vi "Recalculation_Monitor - 3 SC.vi"(0 "Alpha":dbl(slide)=0.17500000000000002 step=0.005 scale=0.0..1.0, 1 "Message 1":string="Lorem ipsum dolor sit amet, consetetur sadipscing elitr, sed diam nonumy eirmod tempor invidunt ut labore et dolore magna aliquyam erat, sed diam volu", 2 "Message 2":string="ptua. At vero eos et accusam et justo duo dolores et ea rebum. Stet clita kasd gubergren, no sea takimata sanctus est Lorem ipsum dolor sit amet. Lore", 3 "Alpha old":dbl(slide)=0.17500000000000002 step=0.005 scale=0.0..1.0, 4 "Message 1 old":string="Lorem ipsum dolor sit amet, consetetur sadipscing elitr, sed diam nonumy eirmod tempor invidunt ut labore et dolore magna aliquyam erat, sed diam volu", 5 "Message 2 old":string="ptua. At vero eos et accusam et justo duo dolores et ea rebum. Stet clita kasd gubergren, no sea takimata sanctus est Lorem ipsum dolor sit amet. Lore", 6 "Beta/Alpha":dbl(slide)=0.17500000000000002 step=0.005 scale=0.0..1.0, 8 "Beta/Alpha old":dbl(slide)=0.17500000000000002 step=0.005 scale=0.0..1.0) -> (14 "Recalculate?":bool, 15 "Recalculate SIG":bool, 16 "Recalculate OFDM":bool)   [LabVIEW 2022 SP3]
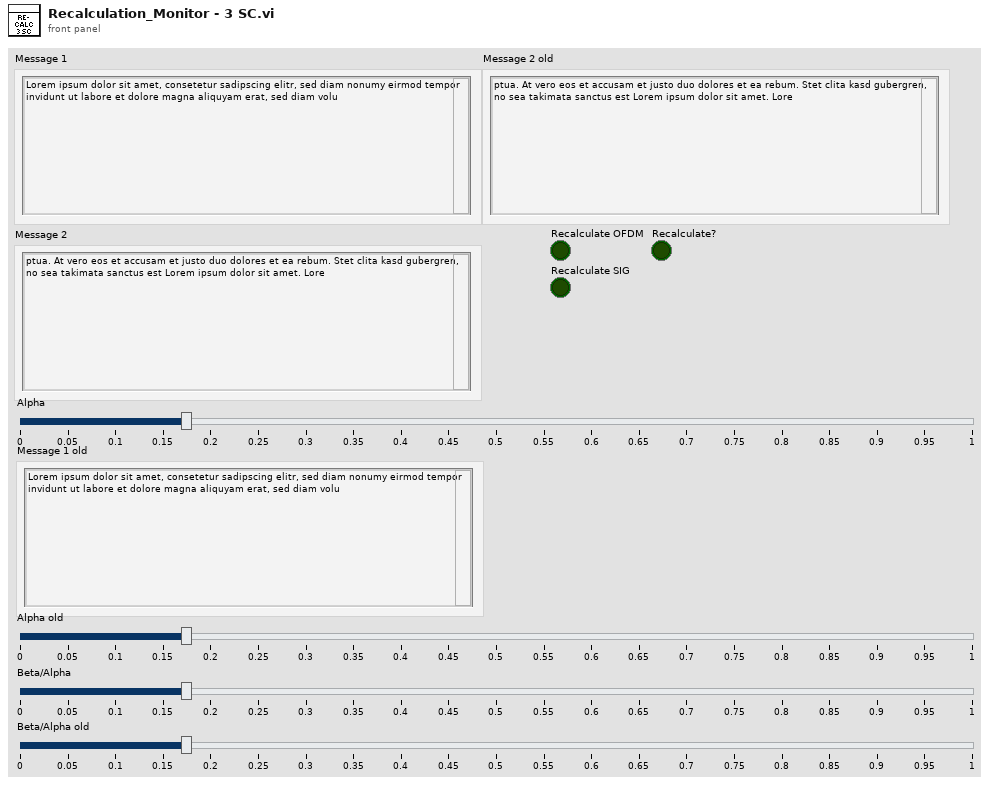
[diagram p1: front panel]
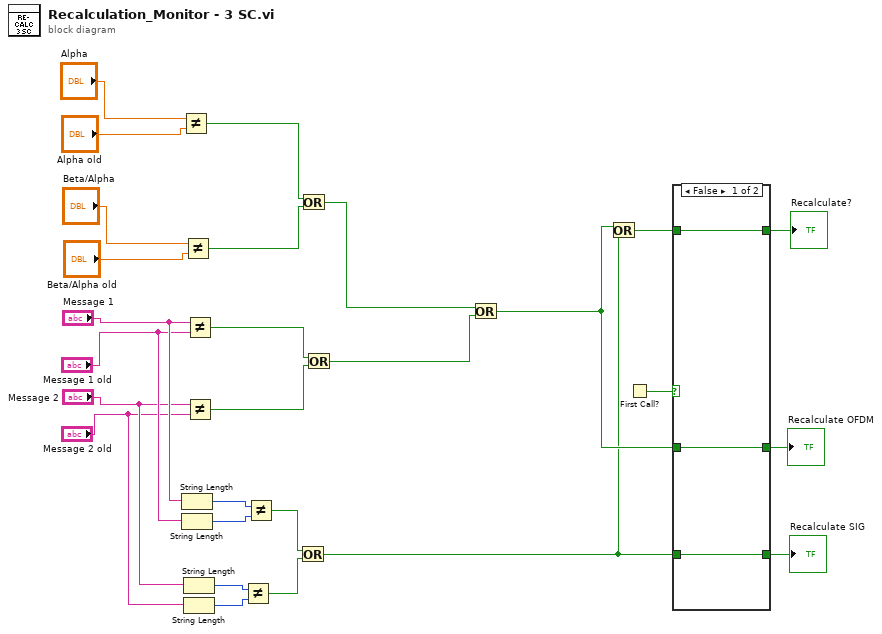
[diagram p0: block diagram]
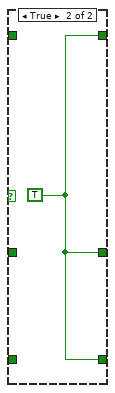
[diagram p2: hidden frame]
diagram:
  n1 = Not Equal?(x="Alpha", y="Alpha old") -> (x != y?=w3:bool)
  n2 = String Length(string="Message 1") -> (length=w19:i32)
  n3 = String Length(string="Message 1 old") -> (length=w18:i32)
  n4 = Not Equal?(x="Beta/Alpha", y="Beta/Alpha old") -> (x != y?=w2:bool)
  n5 = String Length(string="Message 2") -> (length=w17:i32)
  n6 = String Length(string="Message 2 old") -> (length=w16:i32)
  n7 = Not Equal?(x="Message 1", y="Message 1 old") -> (x != y?=w25:bool)
  n8 = Not Equal?(x="Message 2", y="Message 2 old") -> (x != y?=w24:bool)
  n9 = Not Equal?(x=w17, y=w16) -> (x != y?=w14:bool)
  n10 = Not Equal?(x=w19, y=w18) -> (x != y?=w15:bool)
  n11 = Or(x=w15, y=w14) -> (x .or. y?=w6:bool)
  n12 = Or(x=w3, y=w2) -> (x .or. y?=w1:bool)
  n13 = Or(x=w25, y=w24) -> (x .or. y?=w13:bool)
  n14 = Or(x=w1, y=w13) -> (x .or. y?=w7:bool)
  n15 = Or(x=w7, y=w6) -> (x .or. y?=w8:bool)
  n16 = First Call?() -> (First Call?: T/F=w12:bool)
  n17 = case shown="False" w12 {
    tunnel: [w28 w31] -> w11
    tunnel: [w29 w31] -> w10
    tunnel: [w30 w31] -> w9
    tunnel: w8 -> [w30 _]
    tunnel: w7 -> [w29 _]
    tunnel: w6 -> [w28 _]
    frame False {
    }
    frame True {
      w31 = TRUE
    }
  }
  "Recalculate OFDM" <- w10
  "Recalculate SIG" <- w11
  "Recalculate?" <- w9
